vi "In Place Read 1D Array I16.vi"(8 "error in (no error)":errorcluster, 9 "start index (0)":i64, 10 "values in":i16[](array[numeric]), 11 "pointer in":u64) -> (0 "error out":errorcluster, 2 "values out":i16[](array[numeric]), 3 "pointer out":u64)   [LabVIEW 2013, in "Linux RT IPC.Shared Memory.lvlib"]
uses:
  Linux RT IPC.Shared Memory.lvlib
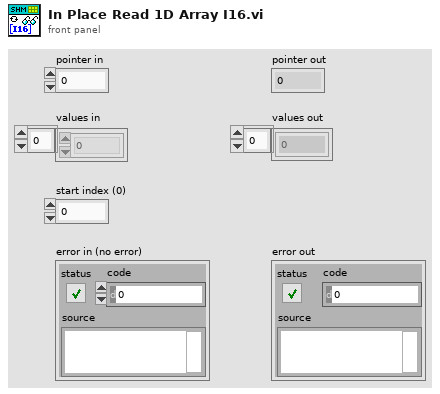
[diagram p1: front panel]
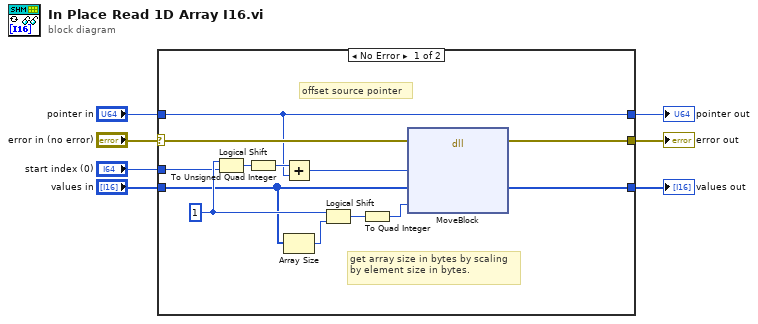
[diagram p0: block diagram]
diagram:
  n1 = case shown="No Error" "error in (no error)" {
    selector: "error in (no error)" -> [w15 w22]
    tunnel: [w14 w22] -> w7
    tunnel: "pointer in" -> [w10 w21]
    tunnel: [w10 w21] -> w4
    tunnel: "values in" -> [w9 _]
    tunnel: "start index (0)" -> [w13 _]
    tunnel: [w12 _] -> w2
    frame No Error {
      w16 = i16 1 ("y")
      # "get array size in bytes by scaling by element size in bytes."
      # "offset source pointer"
      n2 = Logical Shift(y=w16, x=w13) -> (x << y=w19:i64)
      n3 = To Unsigned Quad Integer(1:w19) -> (0:w11:u64)
      n4 = Add(x=w11, y=w10) -> (x+y=w17:u64)
      n5 = Array Size(array=w9) -> (size(s)=w8:i32)
      n6 = Logical Shift(y=w16, x=w8) -> (x << y=w20:i32)
      n7 = To Quad Integer(1:w20) -> (0:w18:i64)
      n8 = dll-call lib="LabVIEW" fn="MoveBlock"(error in=w15, "pointer"=w17, "data"=w9, "size"=w18) -> (error out=w14:errorcluster, "data"=w12:i16[])  [unwired: 5 in, 1 out]
    }
    frame Error {
    }
  }
  "error out" <- w7
  "pointer out" <- w4
  "values out" <- w2
